vi "Time Has Elapsed.vi"(10 "Reset?":bool, 11 "Delay":dbl format="%#_13g") -> (2 "Elapsed Time":dbl, 3 "Elapsed Time Passed?":bool)   [LabVIEW 2020]
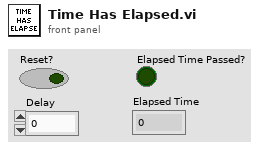
[diagram p1: front panel]
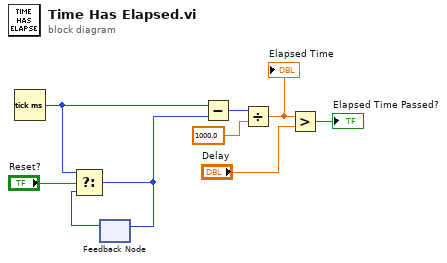
[diagram p0: block diagram]
diagram:
  n1 = Tick Count (ms)() -> (millisecond timer value=w7:u32)
  n2 = feedback #1() -> (w8:u32)  [unwired: 1 in]
  n3 = Select(t=w7, s="Reset?", f=w8) -> (s? t:f=w1:u32)
  n4 = feedback-in #1(w1) -> ()
  n5 = Subtract(x=w7, y=w1) -> (x-y=w4:u32)
  n6 = Divide(x=w4, y=1000.0) -> (x/y=w2:dbl)
  "Elapsed Time" <- w2
  n7 = Greater?(x=w2, y="Delay") -> (0:→"Elapsed Time Passed?":bool)
